vi "处理二维数组.vi"() -> ()   [LabVIEW 2020]
panel:
  out "数组 2":string[][](array[string])=[["a", "b", "c", "d"], ["1", "2", "3", "4"], ["!", "@", "#", "$"]]
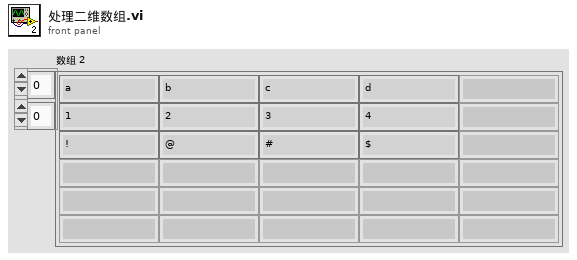
[diagram p1: front panel]
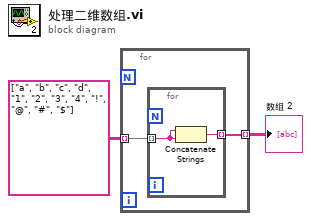
[diagram p0: block diagram]
diagram:
  n1 = for {
    tunnel: string[][] [["a", "b", "c", "d"], ["1", "2", "3", "4"], ["!", "@", "#", "$"]] -> [w4] mode=indexing
    tunnel: [w3] -> w1 mode=indexing
    n2 = for {
      tunnel: w4 -> [w6] mode=indexing
      tunnel: [w5] -> w3 mode=indexing
      n3 = Concatenate Strings(w6, w6) -> (w5:string)
    }
  }
  "数组 2" <- w1
